vi "SPD.Measurments.vi"(5 "Continue":refnum<vi>, 7 "Progress":refnum<vi>, 8 "Error In":errorcluster, 10 "SPD.Meas Setup":T1={"HV_Bias Range"={"Start"=70.0, "Stop"=80.0, "Step"=0.05}, "Strobe_code"={"Start"=0.0, "Stop"=0.0, "Step"=0.0}, "Температура"={"Start"=-45.0, "Stop"=-45.0, "Step"=2.5}} caption="Настройка Измерений", 11 "SPD.Stand Ctrl in":T3 {"spdDeviceSession"."hidSPD.Controller"."HV_bias" format="%#_6p, V"; "spdDeviceSession"."hidSPD.Controller"."TSet" format="%#_6p, DegC"}) -> (0 "Error Out":errorcluster, 1 "pass":bool, 2 "result":string, 3 "SPD.Stand Ctrl out":T3 {"spdDeviceSession"."hidSPD.Controller"."HV_bias" format="%#_6p, V"; "spdDeviceSession"."hidSPD.Controller"."TSet" format="%#_6p, DegC"})   [LabVIEW 2018]
uses:
  <vilib>/Analysis/NI_AALBase.lvlib
  <vilib>/Analysis/1siggen.llb/Ramp Pattern by Delta.vi
  Instruments/SPD HID Interface/hidSPDLibForLabView/LibVIs/hidSPD Controls/hidSPD Device Session.ctl
  Instruments/SPD HID Interface/hidSPDLibForLabView/hidSPDLibForLabView.lvlib
  Instruments/KC705 DevBoard/typedefs/DevB.Session.ctl
  Instruments/KeySight 53230A/typedefs/FreqC.Session.ctl
  Instruments/KeySight 8164B/KeySight 8164B LAN InstrLib/typedefs/KeySight 8164B control.ctl
  Instruments/KeySight 8164B/KeySight 8164B LAN InstrLib.lvlib
  Instruments/LeCroy SDA830/typedefs/LeCroy.Session.ctl
  typedefs/SPD.Stand Ctrl.ctl
  Instruments/SPD HID Interface/hidSPDLibForLabView/LibVIs/hidSPD Controls/hidSPD Controller.ctl
  typedefs/SPD.Events.ctl
  <vilib>/Utility/config.llb/Config Data RefNum.ctl
  <vilib>/Utility/config.llb/NI_LVConfig.lvlib
  SubTests/Measurements/SPD.Test Range.ctl
  SubTests/Measurements/SPD.Grid Meas Setup.ctl
  typedefs/SPD.Meas Result.ctl
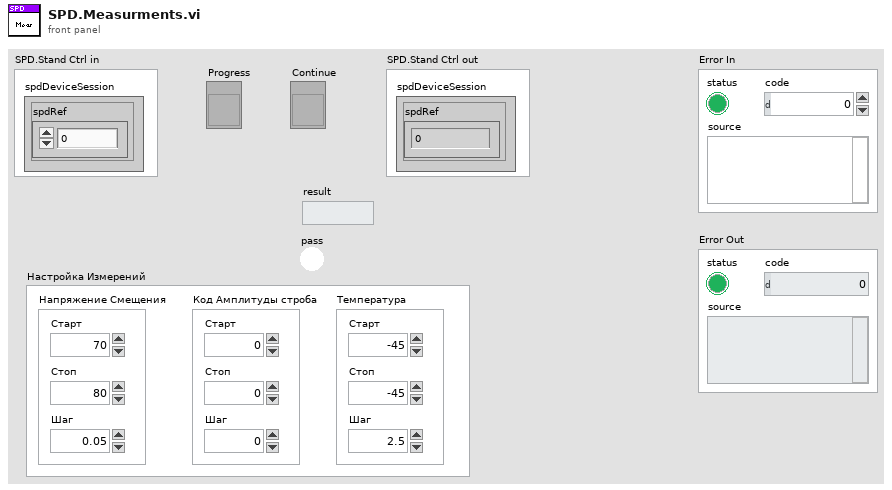
[diagram p1: front panel]
types:
  T1 = typedef "SPD.Grid Meas Setup.ctl" = cluster{"HV_Bias Range":T2, "Strobe_code":T2, "Температура":T2}
  T2 = typedef "SPD.Test Range.ctl" = cluster{"Start":dbl, "Stop":dbl, "Step":dbl}
  T3 = typedef "SPD.Stand Ctrl.ctl" = cluster{"spdDeviceSession":T4, "DevBSession":T6, "FreqCSession":T7, "8164BSession":T8, "LeCroySession":T9, "Events":T10, "configFile":T11, "SPD.Result":T12}
  T4 = typedef "hidSPDLibForLabView.lvlib/hidSPD Device Session.ctl" = cluster{"spdRef":u64, "connected":bool, "spdName":string, "hidSPD.Controller":T5}
  T5 = typedef "hidSPDLibForLabView.lvlib/hidSPD Controller.ctl" = cluster{"TSet":sgl, "HV_bias":sgl, "DDS_stb_code":u16}
  T6 = typedef "DevB.Session.ctl" = cluster{"DevBRef":refnum<visa-resource-name>, "connected":bool}
  T7 = typedef "FreqC.Session.ctl" = cluster{"FreqCRef":refnum<visa-resource-name>, "timeout":dbl, "Gate":dbl, "connected":bool}
  T8 = typedef "KeySight 8164B LAN InstrLib.lvlib/KeySight 8164B control.ctl" = cluster{"Connection ID":refnum<k5>, "Connected":bool, "Info":string, "Slots Info":string[]}
  T9 = typedef "LeCroy.Session.ctl" = cluster{"LeCroySession":refnum<visa-resource-name>, "connected":bool}
  T10 = typedef "SPD.Events.ctl" = cluster{"DCRTest":refnum<user-event>, "Stop":refnum<user-event>}
  T11 = typedef "NI_LVConfig.lvlib/Config Data RefNum.ctl" = refnum<k1>
  T12 = typedef "SPD.Meas Result.ctl" = cluster{"HV_Bias":dbl[][][], "Stb_code":dbl[], "Temprature":dbl[], "Data":dbl[][][][]}
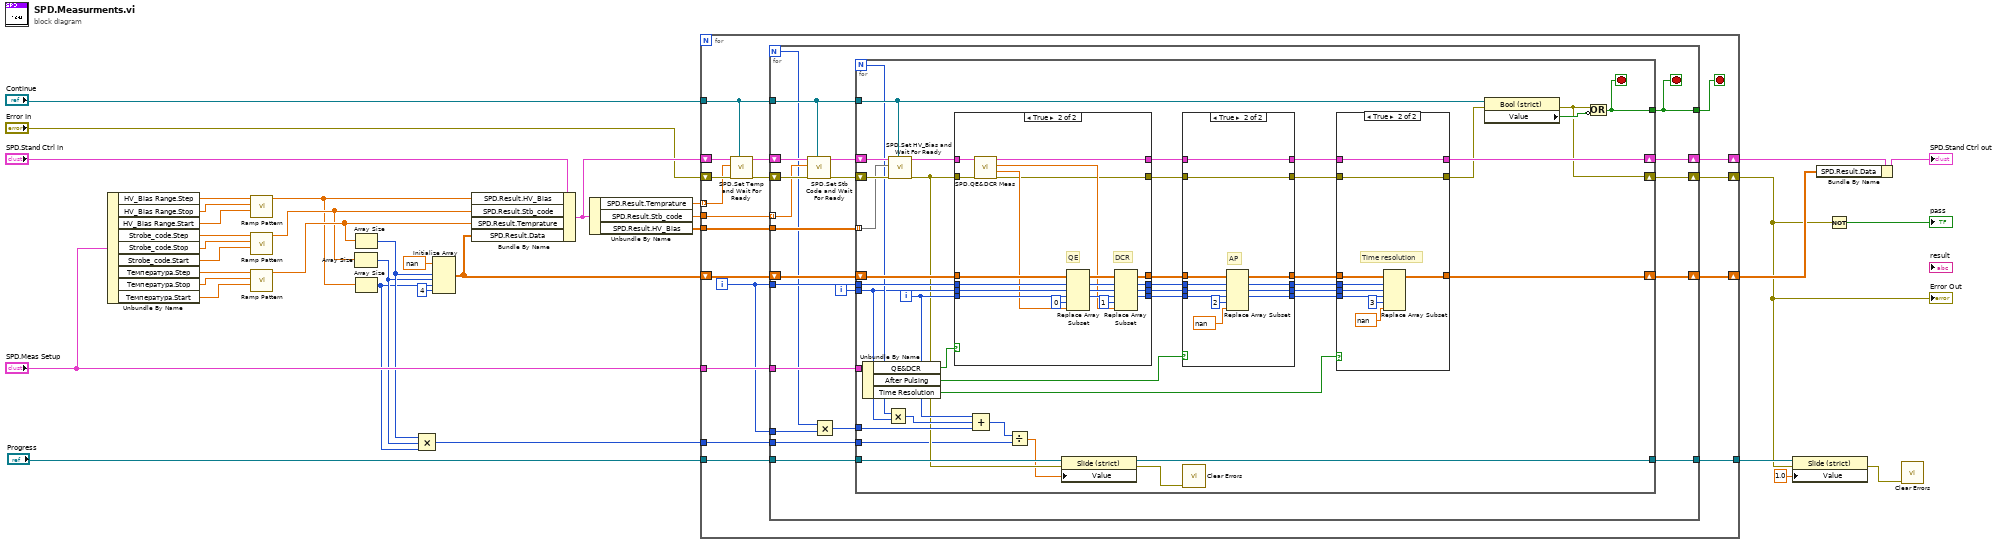
[diagram p0: block diagram]
diagram:
  n1 = Unbundle By Name("SPD.Meas Setup") -> ("HV_Bias Range.Step"=w35:dbl, "HV_Bias Range.Stop"=w34:dbl, "HV_Bias Range.Start"=w33:dbl, "Strobe_code.Step"=w32:dbl, "Strobe_code.Stop"=w31:dbl, "Strobe_code.Start"=w30:dbl, "Температура.Step"=w29:dbl, "Температура.Stop"=w28:dbl, "Температура.Start"=w27:dbl)
  n2 = call-poly <vilib>:"Ramp Pattern.vi"("start"=w33, "end"=w34, "delta"=w35) -> ("Ramp Pattern"=w23:dbl[])  [unwired: 6 in, 2 out]
  n3 = call-poly <vilib>:"Ramp Pattern.vi"("start"=w30, "end"=w31, "delta"=w32) -> ("Ramp Pattern"=w24:dbl[])  [unwired: 6 in, 2 out]
  n4 = call-poly <vilib>:"Ramp Pattern.vi"("start"=w27, "end"=w28, "delta"=w29) -> ("Ramp Pattern"=w25:dbl[])  [unwired: 6 in, 2 out]
  n5 = Array Size(array=w24) -> (size(s)=w8:i32)
  n6 = Array Size(array=w25) -> (size(s)=w9:i32)
  n7 = Array Size(array=w23) -> (size(s)=w7:i32)
  n8 = Compound Arithmetic op=MULTIPLY(w9, w8, w7) -> (w5:i32)
  n9 = Initialize Array(nan ("element"), w9, w8, w7, 4 ("dimension size")) -> (w21:dbl[][][][])
  n10 = Bundle By Name(cluster="SPD.Stand Ctrl in", "SPD.Result.HV_Bias"=w23, "SPD.Result.Stb_code"=w24, "SPD.Result.Temprature"=w25, "SPD.Result.Data"=w21) -> (w19:T3)
  n11 = Unbundle By Name(w19) -> ("SPD.Result.Temprature"=w16:dbl[], "SPD.Result.Stb_code"=w17:dbl[], "SPD.Result.HV_Bias"=w20:dbl[][][])
  n12 = for {
    shift-right: [w50] -> w11
    shift-left: w21 -> [w54]
    tunnel: w20 -> [w53]
    shift-right: [w52] -> w18
    shift-left: w19 -> [w47]
    tunnel: w17 -> [w51]
    tunnel: w16 -> [w44] mode=indexing
    tunnel: "SPD.Meas Setup" -> [w49]
    shift-right: [w48] -> w1
    shift-left: "Error In" -> [w46]
    tunnel: "Continue" -> [w42]
    tunnel: "Progress" -> [w39]
    tunnel: w5 -> [w38]
    tunnel: [w37] -> w4
    i -> [w40]
    stop <- w41 stop-if-true
    n13 = call "SPD.Set Temp and Wait For Ready.vi"("Continue"=w42, "Error In"=w46, "Tset"=w44, "SPD.Stand Ctrl in"=w47) -> ("Error Out"=w45:errorcluster, "SPD.Stand Ctrl out"=w43:T3)  [unwired: 6 in]
    n14 = for {
      N -> [w59]
      shift-right: [w72] -> w50
      shift-left: w54 -> [w74]
      tunnel: w53 -> [w75]
      tunnel: w51 -> [w65] mode=indexing
      shift-right: [w73] -> w52
      shift-left: w43 -> [w69]
      tunnel: w49 -> [w71]
      shift-right: [w70] -> w48
      shift-left: w45 -> [w67]
      tunnel: w42 -> [w64]
      tunnel: w40 -> [w63]
      tunnel: [w61] -> w41
      tunnel: w40 -> [w60]
      tunnel: w39 -> [w57]
      tunnel: w38 -> [w56]
      tunnel: [w55] -> w37
      i -> [w62]
      stop <- w61 stop-if-true
      n15 = call "SPD.Set Stb Code and Wait For Ready.vi"("Continue"=w64, "Error In"=w67, "Strobe code"=w65, "SPD.Stand Ctrl in"=w69) -> ("Error Out"=w66:errorcluster, "SPD.Stand Ctrl out"=w68:T3)  [unwired: 6 in]
      n16 = Multiply(x=w59, y=w60) -> (x*y=w58:i32)
      n17 = for {
        N -> [w87]
        tunnel: w75 -> [w100] mode=indexing
        shift-right: [w106] -> w72
        shift-left: w74 -> [w114]
        shift-right: [w109] -> w73
        shift-left: w68 -> [w103]
        tunnel: w71 -> [w116]
        shift-right: [w89] -> w70
        shift-left: w66 -> [w101]
        tunnel: w64 -> [w92]
        tunnel: w63 -> [w99]
        tunnel: w62 -> [w86]
        tunnel: [w88] -> w61
        tunnel: w58 -> [w83]
        tunnel: w57 -> [w82]
        tunnel: w56 -> [w79]
        tunnel: [w77] -> w55
        i -> [w85]
        stop <- w88 stop-if-true
        n18 = Unbundle By Name(w116) -> ("QE&DCR"=w115:bool, "After Pulsing"=w113:bool, "Time Resolution"=w107:bool)
        n19 = Multiply(x=w87, y=w86) -> (x*y=w84:i32)
        n20 = call "SPD.Set HV_Bias and Wait For Ready.vi"("Continue"=w92, "Error In"=w101, "HV_Bias"=w100, "SPD.Stand Ctrl in"=w103) -> ("Error Out"=w81:errorcluster, "SPD.Stand Ctrl out"=w102:T3)  [unwired: 6 in]
        n21 = case shown="True" w115 {
          tunnel: w114 -> [w147 w163]
          tunnel: w102 -> [w149 w155]
          tunnel: [w149 w150] -> w112
          tunnel: [w147 w160] -> w111
          tunnel: w81 -> [w148 w154]
          tunnel: [w148 w151] -> w105
          tunnel: w99 -> [w146 w158]
          tunnel: w86 -> [w145 w157]
          tunnel: w85 -> [w144 w156]
          tunnel: [w146 w158] -> w98
          tunnel: [w145 w157] -> w97
          tunnel: [w144 w156] -> w96
          frame False {
          }
          frame True {
            # "DCR"
            # "QE"
            n22 = call "SPD.QE&DCR Meas.vi"("Error In"=w154, "SPD.Stand Ctrl in"=w155) -> ("Error Out"=w151:errorcluster, "QE"=w153:dbl, "DCR"=w152:dbl, "SPD.Stand Ctrl out"=w150:T3)  [unwired: 6 in]
            n23 = Replace Array Subset(array=w163, new element=w153, index (dim 0)=w158, index (dim 1)=w157, index (dim 2)=w156, index (dim 3)=0 ("disabled index (col)")) -> (w161:dbl[][][][])
            n24 = Replace Array Subset(array=w161, new element=w152, index (dim 0)=w158, index (dim 1)=w157, index (dim 2)=w156, index (dim 3)=1 ("disabled index (col)")) -> (w160:dbl[][][][])
          }
        }
        n25 = Compound Arithmetic op=ADD(w85, w84, w83) -> (w80:i32)
        n26 = Divide(x=w80, y=w79) -> (x/y=w78:dbl)
        n27 = property class="Slide (strict)"(reference=w82, error in=w81, "Value"=w78) -> (reference out=w77:refnum<vi>, error out=w76:errorcluster)
        n28 = case shown="True" w113 {
          tunnel: w111 -> [w131 w141]
          tunnel: w112 -> [w130 w143]
          tunnel: [w130 w143] -> w110
          tunnel: [w131 w139] -> w108
          tunnel: [w129 w142] -> w104
          tunnel: w105 -> [w129 w142]
          tunnel: w98 -> [w134 w138]
          tunnel: w97 -> [w133 w137]
          tunnel: w96 -> [w132 w136]
          tunnel: [w134 w138] -> w95
          tunnel: [w133 w137] -> w94
          tunnel: [w132 w136] -> w93
          frame False {
          }
          frame True {
            # "AP"
            n29 = Replace Array Subset(array=w141, new element=nan ("element"), index (dim 0)=w138, index (dim 1)=w137, index (dim 2)=w136, index (dim 3)=2 ("disabled index (col)")) -> (w139:dbl[][][][])
          }
        }
        n30 = call <vilib>:"Clear Errors.vi"("error in (no error)"=w76) -> ()  [unwired: 5 in, 2 out]
        n31 = case shown="True" w107 {
          tunnel: w108 -> [w117 w126]
          tunnel: w110 -> [w119 w128]
          tunnel: [w119 w128] -> w109
          tunnel: [w117 w125] -> w106
          tunnel: [w118 w127] -> w91
          tunnel: w104 -> [w118 w127]
          tunnel: w95 -> [_ w124]
          tunnel: w94 -> [_ w123]
          tunnel: w93 -> [_ w122]
          frame False {
          }
          frame True {
            # "Time resolution"
            n32 = Replace Array Subset(array=w126, new element=nan ("element"), index (dim 0)=w124, index (dim 1)=w123, index (dim 2)=w122, index (dim 3)=3 ("disabled index (col)")) -> (w125:dbl[][][][])
          }
        }
        n33 = property class="Bool (strict)"(reference=w92, error in=w91) -> (error out=w89:errorcluster, "Value"=w90:bool)  [unwired: 1 out]
        n34 = Compound Arithmetic op=OR(w89, invert w90) -> (w88:bool)
      }
    }
  }
  "Error Out" <- w1
  n35 = property class="Slide (strict)"(reference=w4, error in=w1, "Value"=1.0) -> (error out=w2:errorcluster)  [unwired: 1 out]
  n36 = Bundle By Name(cluster=w18, "SPD.Result.Data"=w11) -> (→"SPD.Stand Ctrl out":T3)
  n37 = Not(x=w1) -> (.not. x?=→"pass":bool)
  n38 = call <vilib>:"Clear Errors.vi"("error in (no error)"=w2) -> ()  [unwired: 5 in, 2 out]
